vi "AboutGPX.vi"() -> ()   [LabVIEW 2015]
uses:
  ESLSCDLL.dll
panel:
  in  "board_sel":u32=1
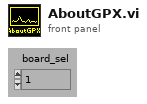
[diagram p1: front panel]
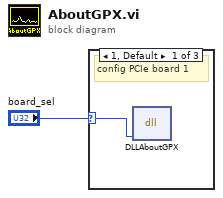
[diagram p0: block diagram]
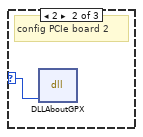
[diagram p2: hidden frame]
diagram:
  n1 = case shown="1, Default" "board_sel" {
    selector: "board_sel" -> [w2 w3 _]
    frame 1, Default {
      # "config PCIe board 1"
      n2 = dll-call lib="C:/Users/flori/Nextcloud/Dokumente/Stresing/Windows/lv64/board.vis/ESLSCDLL.dll" fn="DLLAboutGPX" ("lwlscdll.dll:DLLWriteLongS0")("drv"=w2) -> ()  [unwired: 5 in, 2 out]
    }
    frame 2 {
      # "config PCIe board 2"
      n3 = dll-call lib="C:/Users/flori/Nextcloud/Dokumente/Stresing/Windows/lv64/board.vis/ESLSCDLL.dll" fn="DLLAboutGPX" ("lwlscdll.dll:DLLWriteLongS0")("drv"=w3) -> ()  [unwired: 5 in, 2 out]
    }
    frame 3 {
      # "config both PCIe boards"
    }
  }
